vi "IT8900A-E Series Run Constant Current Transient.vi"() -> ()   [LabVIEW 2015]
uses:
  <instrlib>/IT8900/IT8900A-E.lvlib
panel:
  in  "B Level Value (2)":dbl=2.0 min=0.0 max=7500.0 step=1.0 format="%.4f"
  in  "A Level Value (1)":dbl=1.0 min=0.0 max=7500.0 step=1.0 format="%.4f"
  in  "A Width (1)":dbl=1.0 min=0.0 max=120.0 step=1.0 format="%#.3f"
  in  "B Width (1)":dbl=1.0 min=0.0 max=120.0 step=1.0 format="%#.3f"
  in  "?":bool
  in  "Serial Configuration":cluster{"Baud Rate":u32}={"Baud Rate"=9600} {"Baud Rate" items=["300"=300, "600"=600, "1200"=1200, "2400"=2400, "4800"=4800, "9600"=9600, "19200"=19200]}
  in  "VISA resource name":refnum<visa-resource-name>
  # "ohms"
  # "ohms"
  # "s"
  # "s"
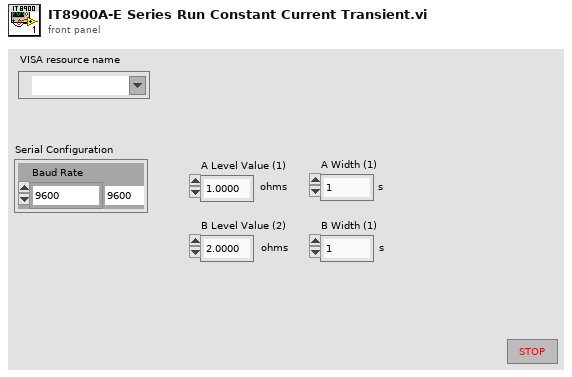
[diagram p1: front panel]
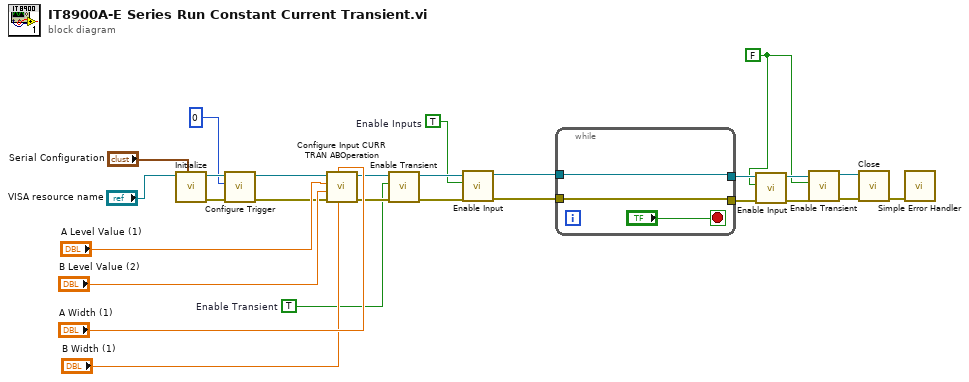
[diagram p0: block diagram]
diagram:
  w6 = FALSE
  w14 = TRUE  # Enable Inputs
  w15 = TRUE  # Enable Transient
  n1 = call <instrlib>:"Initialize.vi"("Serial Configuration"="Serial Configuration", "VISA resource name"="VISA resource name") -> ("error out"=w25:errorcluster, "VISA resource name out"=w24:refnum<visa-resource-name>)  [unwired: 8 in]
  n2 = call <instrlib>:"Configure Trigger.vi"("error in (no error)"=w25, "Trigger Source 0:BUS"=0, "VISA resource name"=w24) -> ("error out"=w4:errorcluster, "VISA resource name out"=w5:refnum<visa-resource-name>)  [unwired: 7 in]
  n3 = call <instrlib>:"Configure Input CURR TRAN ABOperation.vi"("B Width (1)"="B Width (1)", "A Width (1)"="A Width (1)", "error in (no error)"=w4, "B Level Value (2)"="B Level Value (2)", "A Level Value (1)"="A Level Value (1)", "VISA resource name"=w5) -> ("error out"=w18:errorcluster, "VISA resource name out"=w19:refnum<visa-resource-name>)  [unwired: 4 in]
  n4 = call <instrlib>:"Enable Transient.vi"("error in (no error)"=w18, "Enable TRANsient"=w15, "VISA resource name"=w19) -> ("error out"=w16:errorcluster, "VISA resource name out"=w17:refnum<visa-resource-name>)  [unwired: 7 in]
  n5 = call <instrlib>:"Enable Input.vi"("error in (no error)"=w16, "Enable Input"=w14, "VISA resource name"=w17) -> ("error out"=w2:errorcluster, "VISA resource name out"=w3:refnum<visa-resource-name>)  [unwired: 7 in]
  n6 = while {
    tunnel: w3 -> [w29]
    tunnel: w2 -> [w28]
    tunnel: [w29] -> w8
    tunnel: [w28] -> w7
    stop <- "?" stop-if-true
  }
  n7 = call <instrlib>:"Enable Input.vi"("error in (no error)"=w7, "Enable Input"=w6, "VISA resource name"=w8) -> ("error out"=w9:errorcluster, "VISA resource name out"=w10:refnum<visa-resource-name>)  [unwired: 7 in]
  n8 = call <instrlib>:"Enable Transient.vi"("error in (no error)"=w9, "Enable TRANsient"=w6, "VISA resource name"=w10) -> ("error out"=w11:errorcluster, "VISA resource name out"=w12:refnum<visa-resource-name>)  [unwired: 7 in]
  n9 = call <instrlib>:"Close.vi"("error in (no error)"=w11, "VISA resource name"=w12) -> ("error out"=w13:errorcluster)  [unwired: 9 in]
  n10 = call <vilib>:"Simple Error Handler.vi"("error in (no error)"=w13) -> ()  [unwired: 4 in, 5 out]
